vi "IHL_Wait for Inspect Range Helper.vi"(8 "error in (no error)":errorcluster, 10 "Inspect Helper Loop Data":T1={"IHL State"=enum."Init", "Timeout"=-1, "Loop Count"=0, "Start Sample No."=0, "No. Samples"=0, "Collecting Data"=FALSE, "Scan Complete"=FALSE, "Inspect Status "={"Ready"=FALSE, "Inspecting"=FALSE, "Cancel"=FALSE}, "Status"=0, "Encoder Count"=0, "PosToStartScan"=50800, "ScanLength"=50800, "MaxSamples"=50800, "PosToEndScan"=0, "data value reference"=refnum, "Block Cnt notifier out"=refnum, "EventLog"=refnum}, 11 "Message Queue in":refnum<class "Delacor_lib_QMH_Message Queue.lvclass">) -> (0 "error out":errorcluster, 2 "Inspect Helper Loop Data out":T1={"IHL State"=enum."Init", "Timeout"=0, "Loop Count"=0, "Start Sample No."=0, "No. Samples"=0, "Collecting Data"=FALSE, "Scan Complete"=FALSE, "Inspect Status "={"Ready"=FALSE, "Inspecting"=FALSE, "Cancel"=FALSE}, "Status"=0, "Encoder Count"=0, "PosToStartScan"=50800, "ScanLength"=50800, "MaxSamples"=50800, "PosToEndScan"=0, "data value reference"=refnum, "Block Cnt notifier out"=refnum, "EventLog"=refnum})   [LabVIEW 2015, in "Tool Module.lvlib"]
doc: "<b>Note:</b> This VI was modified by the <b>Validate DQMH Module</b> tool to turn off automatic error handling."
uses:
  Tool Module.lvlib
  _IHL Data Cluster--typedef.ctl
  QC-X App/Libraries/Event Logger Library/Event Log/EventLog.lvclass
  _IHL SM Enum--typedef.ctl
  _IHL Status Update Cluster--typedef.ctl
  <vilib>/Delacor/Delacor QMH/Libraries/Message Queue_class/Delacor_lib_QMH_Message Queue.lvclass
  <vilib>/Delacor/Delacor QMH/Libraries/Message Queue_class/Delacor_lib_QMH_Message Queue.lvclass/Delacor_lib_QMH_Message Queue.ctl
  <vilib>/Delacor/Delacor QMH/Libraries/Message Queue_class/Delacor_lib_QMH_Enqueue Message (Single).vi
  ToolModGLOB.vi
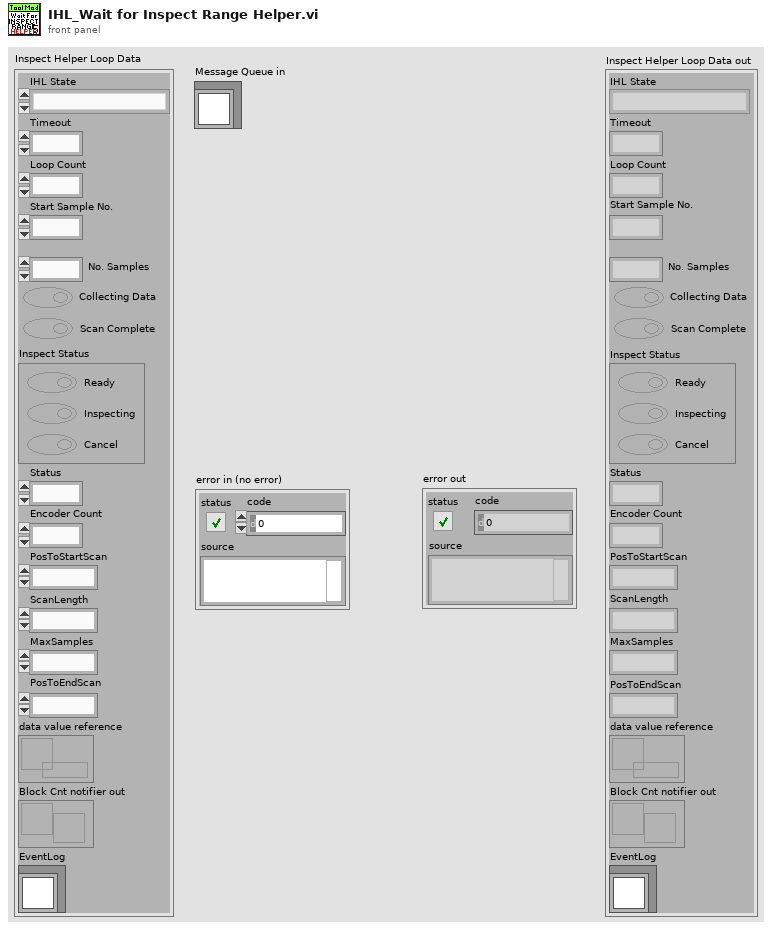
[diagram p1: front panel]
types:
  T1 = typedef "Tool Module.lvlib/_IHL Data Cluster--typedef.ctl" = cluster{"IHL State":T2, "Timeout":i32, "Loop Count":i32, "Start Sample No.":u32, "No. Samples":i32, "Collecting Data":bool, "Scan Complete":bool, "Inspect Status ":T3, "Status":u16, "Encoder Count":i32, "PosToStartScan":i32, "ScanLength":i32, "MaxSamples":i32, "PosToEndScan":i32, "data value reference":refnum<data-value>, "Block Cnt notifier out":refnum<notifier>, "EventLog":refnum<class "EventLog.lvclass">}
  T2 = typedef "Tool Module.lvlib/_IHL SM Enum--typedef.ctl" = enum16{"Init", "Set Motion Speed", "Move To Scan Start", "Wait for Motion Out", "Wait for Start Pos", "Inspect: START", "Wait for Motion IN", "Wait for Inspect Range", "Inspecting", "Inspect: STOP"}
  T3 = typedef "Tool Module.lvlib/_IHL Status Update Cluster--typedef.ctl" = cluster{"Ready":bool, "Inspecting":bool, "Cancel":bool}
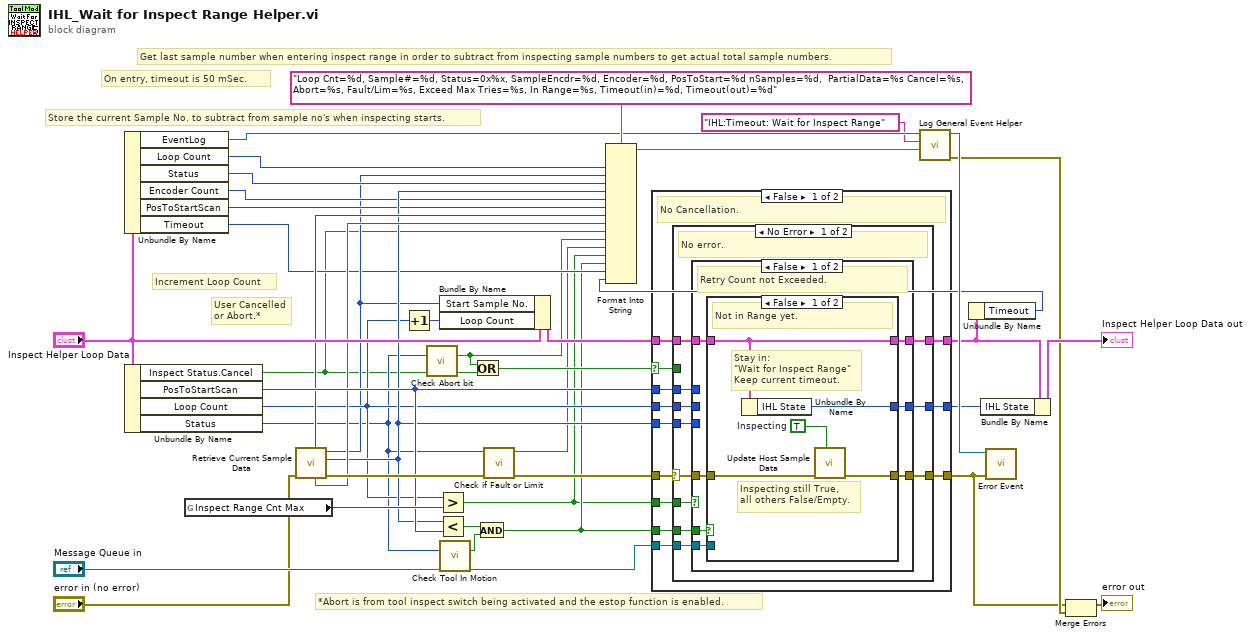
[diagram p0: block diagram]
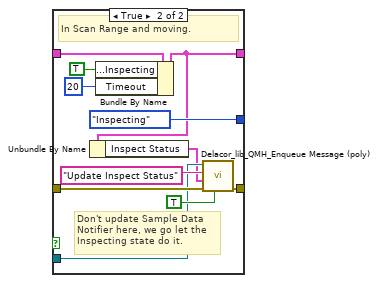
[diagram p2: hidden frame]
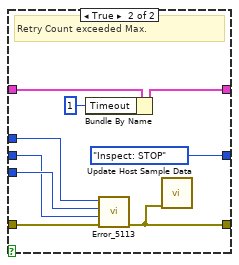
[diagram p3: hidden frame]
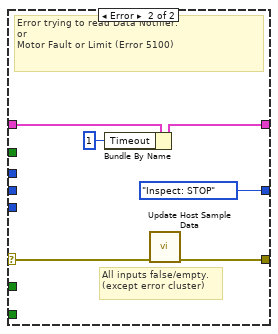
[diagram p4: hidden frame]
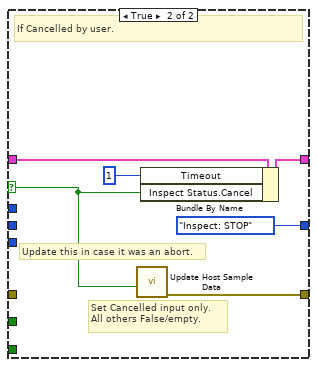
[diagram p5: hidden frame]
diagram:
  # "Get last sample number when entering inspect range in order to subtract from inspecting sample numbers to get actual total sample numbers."
  # "*Abort is from tool inspect switch being activated and the estop function is enabled."
  # "User Cancelled\nor Abort.*"
  # "Store the current Sample No. to subtract from sample no's when inspecting starts."
  # "On entry, timeout is 50 mSec."
  # "Increment Loop Count"
  n1 = Unbundle By Name("Inspect Helper Loop Data") -> ("EventLog"=w20:refnum<class "EventLog.lvclass">, "Loop Count"=w24:i32, "Status"=w23:u16, "Encoder Count"=w22:i32, "PosToStartScan"=w21:i32, "Timeout"=w9:i32)
  n2 = Unbundle By Name("Inspect Helper Loop Data") -> ("Inspect Status.Cancel"=w8:bool, "PosToStartScan"=w30:i32, "Loop Count"=w14:i32, "Status"=w11:u16)
  n3 = global read "ToolModGLOB.vi" "Inspect Range Cnt Max"() -> (w33:i32)
  n4 = call "Retrieve Current Sample Data.vi"("error in (no error)"="error in (no error)") -> ("error out"=w34:errorcluster, "Encoder Out"=w27:i32, "Last Sample No."=w12:u32, "Partial Data"=w28:bool, "nSamples"=w29:u32)  [unwired: 5 in, 1 out]
  n5 = Increment(x=w14) -> (x+1=w13:i32)
  n6 = call "Check Abort bit.vi"("Status Byte"=w11) -> ("Abort?"=w7:bool)  [unwired: 14 in]
  n7 = Greater?(x=w14, y=w33) -> (0:w5:bool)
  n8 = Less?(x=w27, y=w30) -> (x < y?=w31:bool)
  n9 = Bundle By Name(cluster="Inspect Helper Loop Data", "Start Sample No."=w12, "Loop Count"=w13) -> (w35:T1)
  n10 = call "Check Tool In Motion.vi"("Status Byte"=w11) -> ("Tool In Motion?"=w32:bool)  [unwired: 14 in]
  n11 = Or(x=w7, y=w8) -> (x .or. y?=w10:bool)
  n12 = And(x=w31, y=w32) -> (x .and. y?=w6:bool)
  n13 = call "Check if Fault or Limit.vi"("error in (no error)"=w34, "Status In"=w11) -> ("error out"=w25:errorcluster, "Fault or Limit"=w4:bool)  [unwired: 8 in]
  n14 = case shown="False" w10 {
    selector: w10 -> [w41 w101]
    tunnel: [w51 _IHL_SM_Enum--typedef."Inspect: STOP" ("Inspect State")] -> w15
    tunnel: [w52 w102] -> w1
    tunnel: w5 -> [w50 _]
    tunnel: w6 -> [w49 _]
    tunnel: w30 -> [w48 _]
    tunnel: w27 -> [w47 _]
    tunnel: w14 -> [w46 _]
    tunnel: w35 -> [w45 w105]
    tunnel: [w44 w104] -> w3
    tunnel: w25 -> [w43 _]
    tunnel: "Message Queue in" -> [w42 _]
    frame False {
      # "No Cancellation."
      n15 = case shown="No Error" w43 {
        selector: w43 -> [w54 w96]
        tunnel: [w63 w95] -> w52
        tunnel: [w62 _IHL_SM_Enum--typedef."Inspect: STOP" ("Inspect State")] -> w51
        tunnel: w50 -> [w61 _]
        tunnel: w49 -> [w60 _]
        tunnel: w48 -> [w59 _]
        tunnel: w47 -> [w58 _]
        tunnel: w46 -> [w57 _]
        tunnel: w45 -> [w56 w99]
        tunnel: [w55 w98] -> w44
        tunnel: w42 -> [w53 _]
        tunnel: w41 -> [_ _]
        frame No Error {
          # "No error."
          n16 = case shown="False" w61 {
            tunnel: [w67 w86] -> w63
            tunnel: [w69 _IHL_SM_Enum--typedef."Inspect: STOP" ("Inspect State")] -> w62
            tunnel: w60 -> [w70 _]
            tunnel: w54 -> [w68 w93]
            tunnel: w59 -> [_ w92]
            tunnel: w58 -> [_ w91]
            tunnel: w57 -> [_ w90]
            tunnel: w56 -> [w66 w89]
            tunnel: [w65 w88] -> w55
            tunnel: w53 -> [w64 _]
            frame False {
              # "Retry Count not Exceeded."
              n17 = case shown="False" w70 {
                tunnel: [w74 _IHL_SM_Enum--typedef."Inspecting" ("Inspect State")] -> w69
                tunnel: w68 -> [w72 w84]
                tunnel: [w73 w84] -> w67
                tunnel: w66 -> [w75 w83]
                tunnel: [w75 w77] -> w65
                tunnel: w64 -> [_ w78]
                frame False {
                  w71 = TRUE  # Inspecting
                  # "Inspecting still True,\nall others False/Empty."
                  # "Stay in:\n\"Wait for Inspect Range\"\nKeep current timeout."
                  # "Not in Range yet."
                  n18 = Unbundle By Name(w75) -> ("IHL State"=w74:T2)
                  n19 = call "Update Host Sample Data.vi"("InspectCycle"=w71, "error in (no error)"=w72) -> ("error out"=w73:errorcluster)  [unwired: 9 in]
                }
                frame True {
                  # "Don't update Sample Data Notifier here, we go let the Inspecting state do it."
                  # "In Scan Range and moving."
                  n20 = Bundle By Name(cluster=w83, "Inspect Status.Inspecting"=TRUE ("Inspecting"), "Timeout"=20) -> (w77:T1)
                  n21 = Unbundle By Name(w77) -> ("Inspect Status"=w76:T3)
                  n22 = call-poly <vilib>:"Delacor_lib_QMH_Enqueue Message (poly).vi"("Priority Message? (F)"=TRUE, "Message Data"=w76, "Message"="Update Inspect Status", "Message Queue in"=w78) -> ()  [unwired: 6 in, 2 out]
                }
              }
            }
            frame True {
              # "Retry Count exceeded Max."
              n23 = Bundle By Name(cluster=w89, "Timeout"=1) -> (w88:T1)
              n24 = call "Error_5113.vi"("error in (no error)"=w93, "Retry count"=w90, "Encoder"=w91, "Target Pos"=w92) -> ("error out"=w86:errorcluster)  [unwired: 7 in]
              n25 = call "Update Host Sample Data.vi"("error in (no error)"=w86) -> ()  [unwired: 10 in, 1 out]
            }
          }
        }
        frame Error {
          # "All inputs false/empty. (except error cluster)"
          # "Error trying to read Data Notifier.\nor\nMotor Fault or Limit (Error 5100)"
          n26 = Bundle By Name(cluster=w99, "Timeout"=1) -> (w98:T1)
          n27 = call "Update Host Sample Data.vi"("error in (no error)"=w96) -> ("error out"=w95:errorcluster)  [unwired: 10 in]
        }
      }
    }
    frame True {
      # "Update this in case it was an abort."
      # "Set Cancelled input only. All others False/empty."
      # "If Cancelled by user."
      n28 = call "Update Host Sample Data.vi"("Cancelled"=w101) -> ("error out"=w102:errorcluster)  [unwired: 10 in]
      n29 = Bundle By Name(cluster=w105, "Timeout"=1, "Inspect Status.Cancel"=w101) -> (w104:T1)
    }
  }
  n30 = Unbundle By Name(w3) -> ("Timeout"=w2:i32)
  n31 = Format Into String(format string="Loop Cnt=%d, Sample#=%d, Status=0x%x, SampleEncdr=%d, Encoder=%d, PosToStart=%d nSamples=%d,  PartialData=%s Cancel=%s, Abort=%s, Fault/Lim=%s, Exceed Max Tries=%s, In Range=%s, Timeout(in)=%d, Timeout(out)=%d", w24, w12, w23, w27, w22, w21, w29, w28, w8, w7, w4, w5, w6, w9, w2) -> (resulting string=w17:string)  [unwired: 2 in, 1 out]
  n32 = call "Log General Event Helper.vi"("Payload"=w17, "State Info"="IHL:Timeout: Wait for Inspect Range", "EventLog in"=w20) -> ("error out"=w18:errorcluster, "EventLog out"=w19:refnum<class "EventLog.lvclass">)  [unwired: 7 in]
  n33 = Bundle By Name(cluster=w3, "IHL State"=w15) -> (→"Inspect Helper Loop Data out":T1)
  n34 = call "Error Event.vi"("error in (no error)"=w1, "EventLog ref"=w19) -> ()  [unwired: 8 in, 2 out]
  n35 = Merge Errors(w1, w18) -> (→"error out":errorcluster)
